vi "Init.vi"(10 "Front Panel Window:State":T1(ring)) -> (3 "Set Panel State Msg Strategy out":refnum<class "Set Panel State Msg Strategy.lvclass">)   [LabVIEW 2021, in "Set Panel State Msg Strategy.lvlib" / "Set Panel State Msg Strategy.lvclass"]
uses:
  Set Panel State Msg Strategy.lvclass
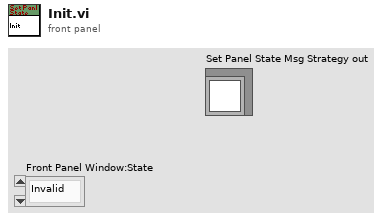
[diagram p1: front panel]
types:
  T1 = enum32{"Invalid", "Standard", "Closed", "Hidden", "Minimized", "Maximized"}
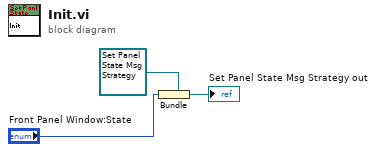
[diagram p0: block diagram]
diagram:
  n1 = Bundle "Bundle"(cluster=refnum<class "Set Panel State Msg Strategy.lvclass"> refnum ("Panel Open Msg Strategy out"), "Front Panel Window:State") -> (→"Set Panel State Msg Strategy out":refnum<class "Set Panel State Msg Strategy.lvclass">)
